vi "Position Numeric Keys.vi"(8 "error in (no error)":errorcluster, 10 "Keys":refnum<vi>[][](array[refnum]), 11 "Input field":refnum<vi>) -> (0 "error out":errorcluster)   [LabVIEW 2014]
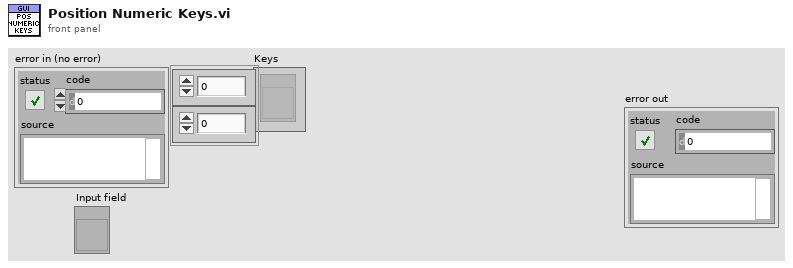
[diagram p1: front panel]
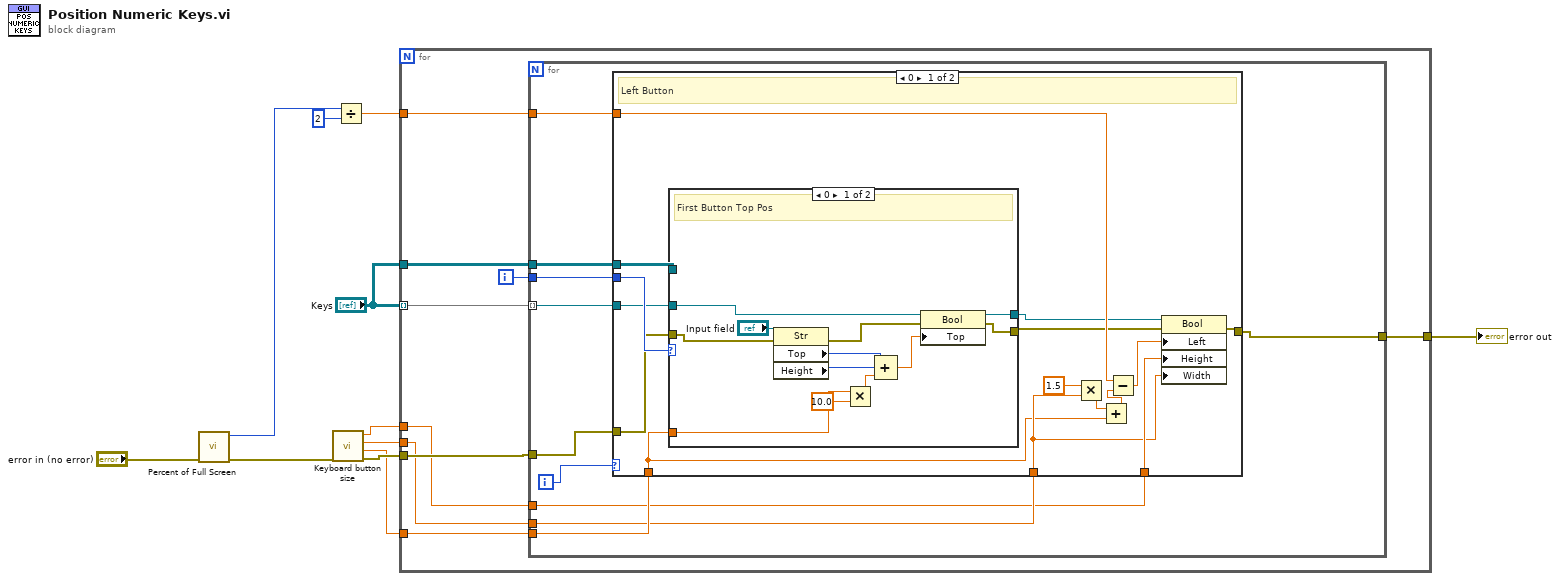
[diagram p0: block diagram]
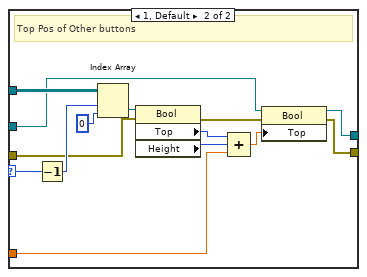
[diagram p2: hidden frame]
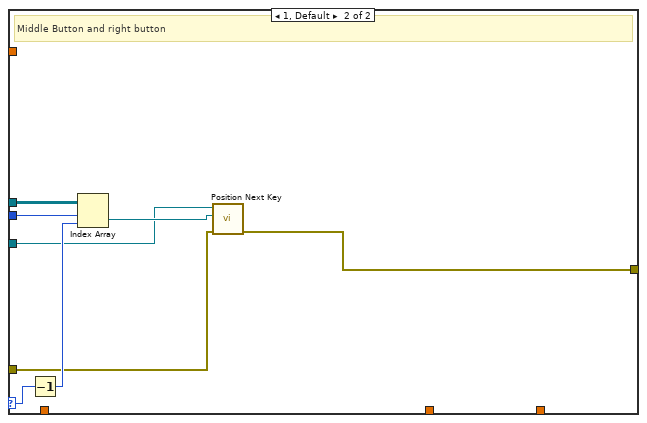
[diagram p3: hidden frame]
diagram:
  n1 = call "Percent of Full Screen.vi"("error in (no error)"="error in (no error)") -> ("error out"=w6:errorcluster, "Right"=w5:i16)  [unwired: 8 in, 1 out]
  n2 = call "Keyboard button size.vi"("error in (no error)"=w6) -> ("error out"=w10:errorcluster, "Key Spacing"=w7:dbl, "Key Width"=w8:dbl, "Key Height"=w9:dbl)  [unwired: 7 in]
  n3 = Divide(x=w5, y=i16 2) -> (x/y=w3:dbl)
  n4 = for {
    tunnel: "Keys" -> [w20] mode=indexing
    tunnel: "Keys" -> [w18]
    tunnel: w10 -> [w17]
    tunnel: w9 -> [w16]
    tunnel: w8 -> [w15]
    tunnel: w7 -> [w14]
    tunnel: w3 -> [w13]
    tunnel: [w12] -> w1
    i -> [w19]
    n5 = for {
      tunnel: w20 -> [w28] mode=indexing
      tunnel: w19 -> [w29]
      tunnel: w18 -> [w26]
      tunnel: w17 -> [w27]
      tunnel: w16 -> [w22]
      tunnel: w15 -> [w23]
      tunnel: w14 -> [w25]
      tunnel: w13 -> [w24]
      tunnel: [w21] -> w12
      i -> [w30]
      n6 = case shown="0" w30 {
        selector: w30 -> [_ w77]
        tunnel: w29 -> [w45 w78]
        tunnel: w28 -> [w44 w73]
        tunnel: w27 -> [w43 w75]
        tunnel: w26 -> [w42 w79]
        tunnel: w25 -> [w32 _]
        tunnel: [w39 w72] -> w21
        tunnel: w24 -> [w40 _]
        tunnel: w23 -> [w34 _]
        tunnel: w22 -> [w35 _]
        frame 0 {
          # "Left Button"
          n7 = case shown="0" w45 {
            selector: w45 -> [_ w70]
            tunnel: w44 -> [w57 w62]
            tunnel: w43 -> [w52 w64]
            tunnel: w42 -> [_ w71]
            tunnel: w32 -> [w48 w63]
            tunnel: [w50 w59] -> w36
            tunnel: [w49 w58] -> w37
            frame 0 {
              # "First Button Top Pos"
              n8 = property class="Str"(reference="Input field", error in=w52) -> (error out=w51:errorcluster, "Top"=w55:i32, "Height"=w56:u32)  [unwired: 1 out]
              n9 = Multiply(x=w48, y=10.0) -> (x*y=w46:dbl)
              n10 = Compound Arithmetic op=ADD(w55, w56, w46) -> (w53:dbl)
              n11 = property class="Bool"(reference=w57, error in=w51, "Top"=w53) -> (reference out=w49:refnum<vi>, error out=w50:errorcluster)
            }
            frame 1, Default {
              # "Top Pos of Other buttons"
              n12 = Decrement(x=w70) -> (x-1=w69:i32)
              n13 = Index Array(array=w71, index (row)=w69, index (col)=0 ("disabled index (col)")) -> (element=w67:refnum<vi>)
              n14 = property class="Bool"(reference=w67, error in=w64) -> (error out=w61:errorcluster, "Top"=w66:i32, "Height"=w65:u32)  [unwired: 1 out]
              n15 = Compound Arithmetic op=ADD(w66, w65, w63) -> (w60:dbl)
              n16 = property class="Bool"(reference=w62, error in=w61, "Top"=w60) -> (reference out=w58:refnum<vi>, error out=w59:errorcluster)
            }
          }
          n17 = Multiply(x=1.5, y=w34) -> (x*y=w33:dbl)
          n18 = Add(x=w33, y=w32) -> (x+y=w31:dbl)
          n19 = Subtract(x=w40, y=w31) -> (x-y=w38:dbl)
          n20 = property class="Bool"(reference=w37, error in=w36, "Left"=w38, "Height"=w35, "Width"=w34) -> (error out=w39:errorcluster)  [unwired: 1 out]
        }
        frame 1, Default {
          # "Middle Button and right button"
          n21 = Decrement(x=w77) -> (x-1=w76:i32)
          n22 = Index Array(array=w79, index (row)=w78, index (col)=w76) -> (element=w74:refnum<vi>)
          n23 = call "Position Next Key.vi"("error in (no error)"=w75, "Previous Key"=w74, "Input Key"=w73) -> ("error out"=w72:errorcluster)  [unwired: 8 in]
        }
      }
    }
  }
  "error out" <- w1
